vi "SolenoidActuator.vi"(7 "Action":enum16{"Init", "SetState", "Disable"}(ring), 8 "error in":errorcluster, 9 "Reverse Actuation":bool, 10 "Actuate?":bool, 11 "SolenoidDevRef":T1={"DevStatus"={"status"=FALSE, "code"=0, "source"=""}, "Pneumatics Control Module"=0, "Forward Solenoid Channel"=enum."Invalid", "Reverse Solenoid Channel"=enum."Invalid"}) -> (0 "error out":errorcluster, 3 "SolenoidDevRef out":T1={"DevStatus"={"status"=FALSE, "code"=0, "source"=""}, "Pneumatics Control Module"=0, "Forward Solenoid Channel"=enum."Invalid", "Reverse Solenoid Channel"=enum."Invalid"})   [LabVIEW 2016]
doc: "Controls a single solenoid. It has the following actions:\n-Init: takes a reference to a single solenoid and stores it in a shift register so that the reference does not need to be passed again. Also takes a boolean for default position: if default position is false (the \"normal\" case), then Off corresponds to the retracted state and On corresponds to the actuated state. If default position is true, then Off corresponds to the *actuated* state and On corresponds to the *retracted* state.\n-SetValue: sets the position of the solenoid. True actuates the solenoid, false retracts it.\n-Disable: sets the solenoid to the retracted position."
uses:
  <vilib>/Rock Robotics/WPI/Solenoid/WPI_SolenoidDevRef.ctl
  <vilib>/Rock Robotics/WPI/Solenoid/WPI_SolenoidChannel.ctl
  <vilib>/Rock Robotics/WPI/Solenoid/WPI_SolenoidValue.ctl
  <vilib>/Rock Robotics/WPI/Solenoid/WPI_SolenoidSetEnum.vi
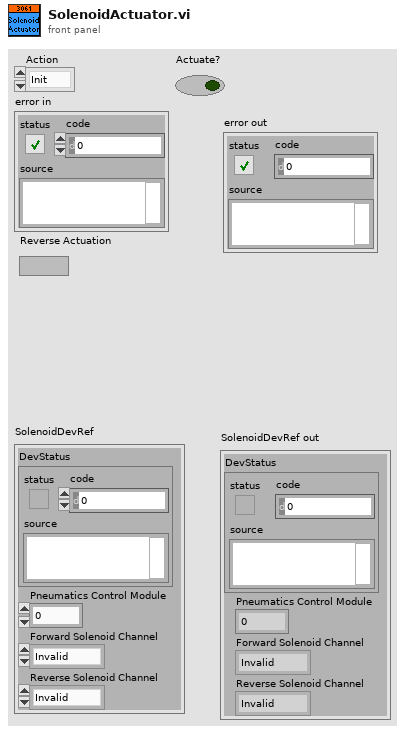
[diagram p1: front panel]
types:
  T1 = typedef "WPI_SolenoidDevRef.ctl" = cluster{"DevStatus":errorcluster, "Pneumatics Control Module":u8, "Forward Solenoid Channel":T2, "Reverse Solenoid Channel":T2}
  T2 = typedef "WPI_SolenoidChannel.ctl" = enum8{"Solenoid 0", "Solenoid 1", "Solenoid 2", "Solenoid 3", "Solenoid 4", "Solenoid 5", "Solenoid 6", "Solenoid 7", "Invalid"}
  T3 = typedef "WPI_SolenoidValue.ctl" = enum16{"Off", "On", "Forward", "Reverse"}
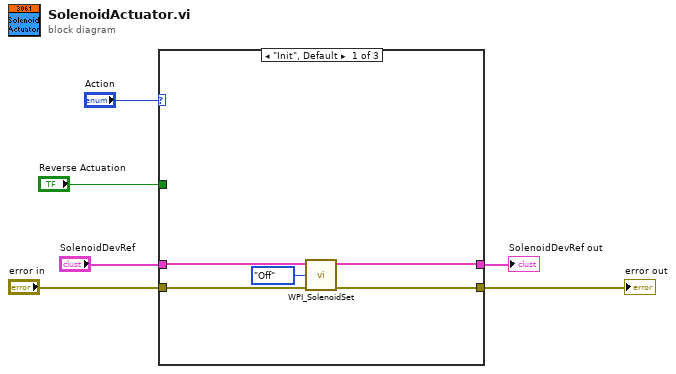
[diagram p0: block diagram]
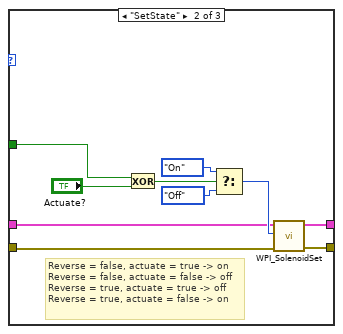
[diagram p2: hidden frame]
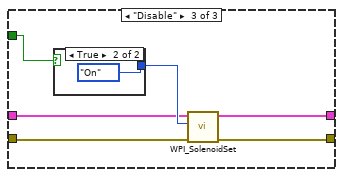
[diagram p3: hidden frame]
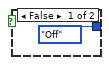
[diagram p4: hidden frame]
diagram:
  n1 = case shown="\"Init\", Default" "Action" {
    tunnel: "SolenoidDevRef" -> [w10 w13 w26]
    tunnel: "error in" -> [w9 w14 w25]
    tunnel: [w8 w15 w24] -> w3
    tunnel: "Reverse Actuation" -> [_ w20 w23]
    tunnel: [w7 w12 w22] -> w1
    frame "Init", Default {
      n2 = call-poly <vilib>:"WPI_SolenoidSet.vi"("error in (no error)"=w9, "Value"=WPI_SolenoidValue."Off", "SolenoidDevRef"=w10) -> ("error out"=w8:errorcluster, "SolenoidDevRef"=w7:T1)  [unwired: 7 in]
    }
    frame "SetState" {
      # "Reverse = false, actuate = true -> on\nReverse = false, actuate = false -> off\nReverse = true, actuate = true -> off\nReverse = true, actuate = false -> on"
      n3 = Exclusive Or(1:"Actuate?", 2:w20) -> (0:w19:bool)
      n4 = Select(t=WPI_SolenoidValue."On" ("Value"), s=w19, f=WPI_SolenoidValue."Off" ("Value")) -> (s? t:f=w16:T3)
      n5 = call-poly <vilib>:"WPI_SolenoidSet.vi"("error in (no error)"=w14, "Value"=w16, "SolenoidDevRef"=w13) -> ("error out"=w15:errorcluster, "SolenoidDevRef"=w12:T1)  [unwired: 7 in]
    }
    frame "Disable" {
      n6 = case shown="True" w23 {
        tunnel: [WPI_SolenoidValue."Off" ("Value") WPI_SolenoidValue."On" ("Value")] -> w27
        frame False {
        }
        frame True {
        }
      }
      n7 = call-poly <vilib>:"WPI_SolenoidSet.vi"("error in (no error)"=w25, "Value"=w27, "SolenoidDevRef"=w26) -> ("error out"=w24:errorcluster, "SolenoidDevRef"=w22:T1)  [unwired: 7 in]
    }
  }
  "error out" <- w3
  "SolenoidDevRef out" <- w1
